vi "Min_UpdateInfo.vi"(8 "error in":errorcluster, 10 "Vibrometer in":T1={"Bandwidth"=10, "High Pass"=0, "Range"=50, "Beam"=TRUE, "Model"="IVS-500", "Version"="1.0302", "Baudrate"="9600", "Autofocus"=FALSE} {"Range" items=["10 mm/s"=1, "20 mm/s"=2, "50 mm/s"=5, "100 mm/s"=10, "200 mm/s"=20, "500 mm/s"=50, "1 m/s"=100, "2 m/s"=200]; "High Pass" items=["Off", "13 Hz", "104 Hz"]; "Bandwidth" items=["1 kHz"=1, "5 kHz"=5, "10 kHz"=10, "25 kHz"=25, "50 kHz"=50, "100 kHz"=100]}, 11 "VISA in":refnum<visa-resource-name>) -> (0 "error out":errorcluster, 1 "Readings":T2={"Temp"=30.2, "Overtemp"=FALSE, "Signal"=8, "Focusing?"=FALSE} {"Signal" scale=0.0..50.0; "Temp" scale=0.0..50.0}, 2 "Vibrometer out":T1={"Bandwidth"=10, "High Pass"=0, "Range"=50, "Beam"=TRUE, "Model"="IVS-500", "Version"="1.0302", "Baudrate"="9600", "Autofocus"=FALSE} {"Range" items=["10 mm/s"=1, "20 mm/s"=2, "50 mm/s"=5, "100 mm/s"=10, "200 mm/s"=20, "500 mm/s"=50, "1 m/s"=100, "2 m/s"=200]; "High Pass" items=["Off", "13 Hz", "104 Hz"]; "Bandwidth" items=["1 kHz"=1, "5 kHz"=5, "10 kHz"=10, "25 kHz"=25, "50 kHz"=50, "100 kHz"=100]}, 3 "VISA out":refnum<visa-resource-name>)   [LabVIEW 2024]
uses:
  <vilib>/Utility/error.llb/Trim Whitespace One-Sided.vi
panel:
  out "comm":cluster{"Sent":string, "Received":string}
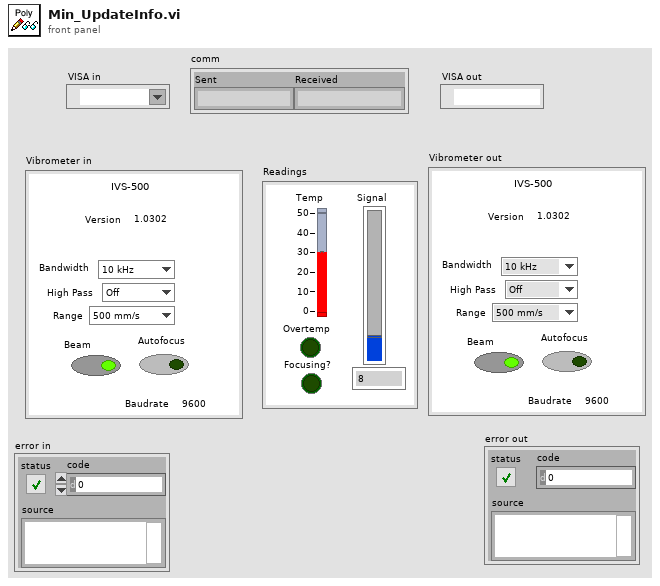
[diagram p1: front panel]
types:
  T1 = cluster{"Bandwidth":u16, "High Pass":u16, "Range":u16, "Beam":bool, "Model":string, "Version":string, "Baudrate":string, "Autofocus":bool}
  T2 = cluster{"Temp":dbl, "Overtemp":bool, "Signal":u8, "Focusing?":bool}
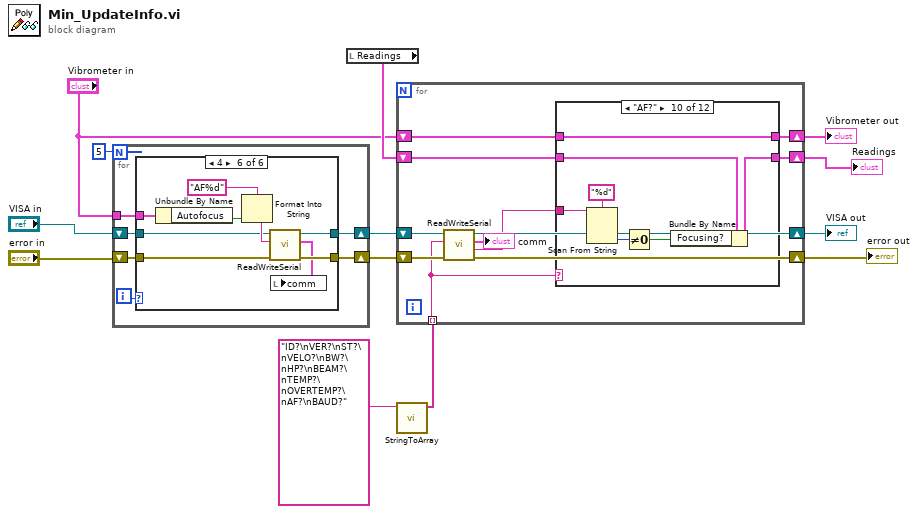
[diagram p0: block diagram]
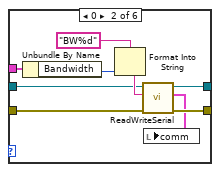
[diagram p3: hidden frame]
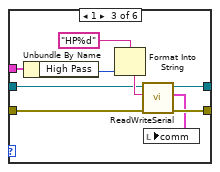
[diagram p4: hidden frame]
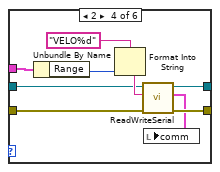
[diagram p5: hidden frame]
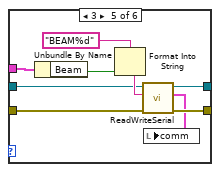
[diagram p6: hidden frame]
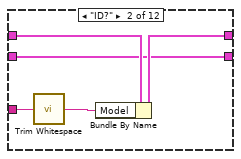
[diagram p8: hidden frame]
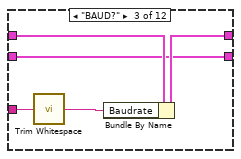
[diagram p9: hidden frame]
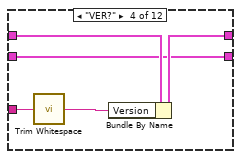
[diagram p10: hidden frame]
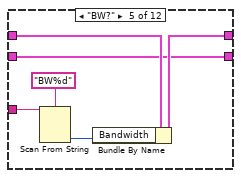
[diagram p11: hidden frame]
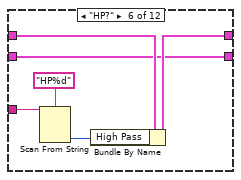
[diagram p12: hidden frame]
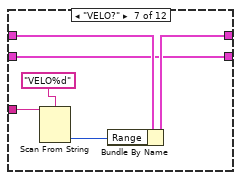
[diagram p13: hidden frame]
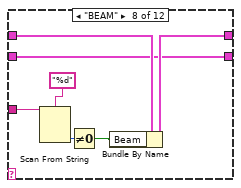
[diagram p14: hidden frame]
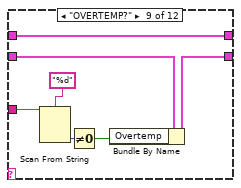
[diagram p15: hidden frame]
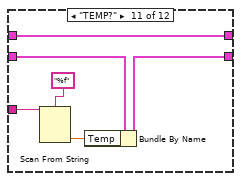
[diagram p16: hidden frame]
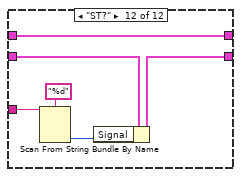
[diagram p17: hidden frame]
diagram:
  n1 = for {
    N: 5 -> [_]
    tunnel: "Vibrometer in" -> [w18]
    shift-right: [w16] -> w3
    shift-left: "VISA in" -> [w17]
    shift-right: [w14] -> w1
    shift-left: "error in" -> [w15]
    i -> [w19]
    n2 = case shown="4" w19 {
      tunnel: w18 -> [_ w30 w39 w48 w57 w66]
      tunnel: w17 -> [w21 w26 w35 w44 w53 w62]
      tunnel: [w21 w25 w34 w43 w52 w61] -> w16
      tunnel: w15 -> [w20 w24 w33 w42 w51 w60]
      tunnel: [w20 w23 w32 w41 w50 w59] -> w14
      frame Default {
      }
      frame 0 {
        n3 = Unbundle By Name(w30) -> ("Bandwidth"=w28:u16)
        n4 = Format Into String(format string="BW%d", w28) -> (resulting string=w27:string)  [unwired: 2 in, 1 out]
        n5 = call "ReadWriteSerial.vi"("error in (no error)"=w24, "cmd"=w27, "VISA Refnum in"=w26) -> ("error out"=w23:errorcluster, "comm"=w22:cluster{"Sent":string, "Received":string}, "VISA Refnum out"=w25:refnum<visa-resource-name>)  [unwired: 5 in, 1 out]
        n6 = local write "comm"(w22) -> ()
      }
      frame 1 {
        n7 = Unbundle By Name(w39) -> ("High Pass"=w37:u16)
        n8 = Format Into String(format string="HP%d", w37) -> (resulting string=w36:string)  [unwired: 2 in, 1 out]
        n9 = call "ReadWriteSerial.vi"("error in (no error)"=w33, "cmd"=w36, "VISA Refnum in"=w35) -> ("error out"=w32:errorcluster, "comm"=w31:cluster{"Sent":string, "Received":string}, "VISA Refnum out"=w34:refnum<visa-resource-name>)  [unwired: 5 in, 1 out]
        n10 = local write "comm"(w31) -> ()
      }
      frame 2 {
        n11 = Unbundle By Name(w48) -> ("Range"=w46:u16)
        n12 = Format Into String(format string="VELO%d", w46) -> (resulting string=w45:string)  [unwired: 2 in, 1 out]
        n13 = call "ReadWriteSerial.vi"("error in (no error)"=w42, "cmd"=w45, "VISA Refnum in"=w44) -> ("error out"=w41:errorcluster, "comm"=w40:cluster{"Sent":string, "Received":string}, "VISA Refnum out"=w43:refnum<visa-resource-name>)  [unwired: 5 in, 1 out]
        n14 = local write "comm"(w40) -> ()
      }
      frame 3 {
        n15 = Unbundle By Name(w57) -> ("Beam"=w55:bool)
        n16 = Format Into String(format string="BEAM%d", w55) -> (resulting string=w54:string)  [unwired: 2 in, 1 out]
        n17 = call "ReadWriteSerial.vi"("error in (no error)"=w51, "cmd"=w54, "VISA Refnum in"=w53) -> ("error out"=w50:errorcluster, "comm"=w49:cluster{"Sent":string, "Received":string}, "VISA Refnum out"=w52:refnum<visa-resource-name>)  [unwired: 5 in, 1 out]
        n18 = local write "comm"(w49) -> ()
      }
      frame 4 {
        n19 = Unbundle By Name(w66) -> ("Autofocus"=w64:bool)
        n20 = Format Into String(format string="AF%d", w64) -> (resulting string=w63:string)  [unwired: 2 in, 1 out]
        n21 = call "ReadWriteSerial.vi"("error in (no error)"=w60, "cmd"=w63, "VISA Refnum in"=w62) -> ("error out"=w59:errorcluster, "comm"=w58:cluster{"Sent":string, "Received":string}, "VISA Refnum out"=w61:refnum<visa-resource-name>)  [unwired: 5 in, 1 out]
        n22 = local write "comm"(w58) -> ()
      }
    }
  }
  n23 = local read "Readings"() -> (w11:T2)
  n24 = call "StringToArray.vi"("write buffer"="ID?\nVER?\nST?\nVELO?\nBW?\nHP?\nBEAM?\nTEMP?\nOVERTEMP?\nAF?\nBAUD?") -> ("Array"=w12:string[])  [unwired: 10 in]
  n25 = for {
    tunnel: w12 -> [w73] mode=indexing
    shift-right: [w77] -> w7
    shift-left: w1 -> [w75]
    shift-right: [w76] -> w8
    shift-left: w3 -> [w74]
    shift-right: [w70] -> w10
    shift-left: "Vibrometer in" -> [w71]
    shift-right: [w68] -> w9
    shift-left: w11 -> [w69]
    n26 = call "ReadWriteSerial.vi"("error in (no error)"=w75, "cmd"=w73, "VISA Refnum in"=w74) -> ("error out"=w77:errorcluster, "Reply"=w72:string, "comm"=→"comm":cluster{"Sent":string, "Received":string}, "VISA Refnum out"=w76:refnum<visa-resource-name>)  [unwired: 5 in]
    n27 = case shown="\"AF?\"" w73 {
      tunnel: w72 -> [_ w84 w89 w94 w100 w106 w112 w119 w126 w133 w139 w145]
      tunnel: w71 -> [w79 w83 w88 w93 w97 w103 w110 w115 w123 w129 w137 w143]
      tunnel: [w79 w82 w87 w92 w96 w102 w108 w114 w123 w129 w137 w143] -> w70
      tunnel: w69 -> [w78 w80 w85 w90 w95 w101 w107 w113 w122 w128 w136 w141]
      tunnel: [w78 w80 w85 w90 w95 w101 w107 w113 w121 w127 w134 w140] -> w68
      frame Default {
      }
      frame "ID?" {
        n28 = call <vilib>:"Trim Whitespace.vi"("string"=w84) -> ("trimmed string"=w81:string)  [unwired: 1 in]
        n29 = Bundle By Name(cluster=w83, "Model"=w81) -> (w82:T1)
      }
      frame "BAUD?" {
        n30 = call <vilib>:"Trim Whitespace.vi"("string"=w89) -> ("trimmed string"=w86:string)  [unwired: 1 in]
        n31 = Bundle By Name(cluster=w88, "Baudrate"=w86) -> (w87:T1)
      }
      frame "VER?" {
        n32 = call <vilib>:"Trim Whitespace.vi"("string"=w94) -> ("trimmed string"=w91:string)  [unwired: 1 in]
        n33 = Bundle By Name(cluster=w93, "Version"=w91) -> (w92:T1)
      }
      frame "BW?" {
        n34 = Scan From String(format string="BW%d", input string=w100) -> (output 1=w98:i32)  [unwired: 3 in, 3 out]
        n35 = Bundle By Name(cluster=w97, "Bandwidth"=w98) -> (w96:T1)
      }
      frame "HP?" {
        n36 = Scan From String(format string="HP%d", input string=w106) -> (output 1=w104:i32)  [unwired: 3 in, 3 out]
        n37 = Bundle By Name(cluster=w103, "High Pass"=w104) -> (w102:T1)
      }
      frame "VELO?" {
        n38 = Scan From String(format string="VELO%d", input string=w112) -> (output 1=w109:i32)  [unwired: 3 in, 3 out]
        n39 = Bundle By Name(cluster=w110, "Range"=w109) -> (w108:T1)
      }
      frame "BEAM" {
        n40 = Scan From String(format string="%d", input string=w119) -> (output 1=w117:i32)  [unwired: 3 in, 3 out]
        n41 = Not Equal To 0?(x=w117) -> (x != 0?=w116:bool)
        n42 = Bundle By Name(cluster=w115, "Beam"=w116) -> (w114:T1)
      }
      frame "OVERTEMP?" {
        n43 = Scan From String(format string="%d", input string=w126) -> (output 1=w124:i32)  [unwired: 3 in, 3 out]
        n44 = Not Equal To 0?(x=w124) -> (x != 0?=w120:bool)
        n45 = Bundle By Name(cluster=w122, "Overtemp"=w120) -> (w121:T2)
      }
      frame "AF?" {
        n46 = Scan From String(format string="%d", input string=w133) -> (output 1=w131:i32)  [unwired: 3 in, 3 out]
        n47 = Not Equal To 0?(x=w131) -> (x != 0?=w130:bool)
        n48 = Bundle By Name(cluster=w128, "Focusing?"=w130) -> (w127:T2)
      }
      frame "TEMP?" {
        n49 = Scan From String(format string="%f", input string=w139) -> (output 1=w135:dbl)  [unwired: 3 in, 3 out]
        n50 = Bundle By Name(cluster=w136, "Temp"=w135) -> (w134:T2)
      }
      frame "ST?" {
        n51 = Scan From String(format string="%d", input string=w145) -> (output 1=w142:i32)  [unwired: 3 in, 3 out]
        n52 = Bundle By Name(cluster=w141, "Signal"=w142) -> (w140:T2)
      }
    }
  }
  "Readings" <- w9
  "VISA out" <- w8
  "error out" <- w7
  "Vibrometer out" <- w10
